vi "FromMonitorZoomOffset.vi"(8 "error in":errorcluster, 10 "Size":T1, 11 "Offset":T1) -> ()   [LabVIEW 2016]
uses:
  <vilib>/Utility/miscctls.llb/LVPointDoubleTypeDef.ctl
  Course Project/support/Message Queue/Message Cluster.ctl
  Course Project/support/Message Queue/Message Queue.lvlib
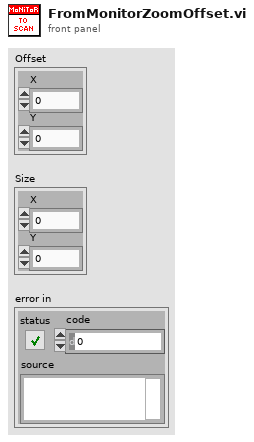
[diagram p1: front panel]
types:
  T1 = typedef "LVPointDoubleTypeDef.ctl" = cluster{"X":dbl, "Y":dbl}
  T2 = typedef "Message Queue.lvlib/Message Cluster.ctl" = cluster{"Message":string, "Données de message":variant}
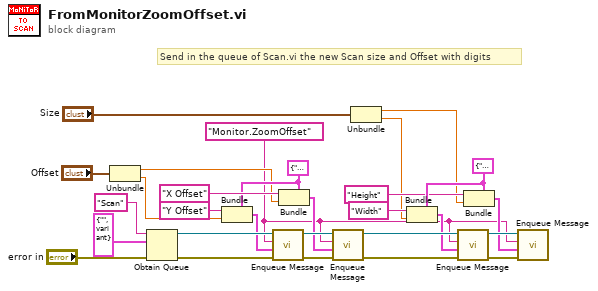
[diagram p0: block diagram]
diagram:
  w28 = cluster{"ControlName":string, "Value":dbl} {"ControlName"="", "Value"=0.0} ("Data")
  w9 = cluster{"ControlName":string, "Value":dbl} {"ControlName"="", "Value"=0.0} ("Data")
  w5 = "Monitor.ZoomOffset" ("Message")
  # "Send in the queue of Scan.vi the new Scan size and Offset with digits"
  n1 = Unbundle("Offset") -> ("X"=w6:dbl, "Y"=w10:dbl)
  n2 = Obtain Queue(name (unnamed)="Scan" ("QueueName"), element data type=T2 {"Message"="", "Données de message"=variant} ("Cluster Message"), error in (no error)="error in") -> (queue out=w26:refnum<queue>, error out=w15:errorcluster)  [unwired: 2 in, 1 out]
  n3 = Bundle(cluster=w9, "ControlName"="Y Offset" ("Message"), "Value"=w10) -> (w8:cluster{"ControlName":string, "Value":dbl})
  n4 = call "Enqueue Message.vi"("error in"=w15, "Data"=w8, "Message"=w5, "Queue"=w26) -> ("error out"=w16:errorcluster, "Queue dup."=w24:refnum<queue>)  [unwired: 6 in]
  n5 = Bundle(cluster=w9, "ControlName"="X Offset" ("Message"), "Value"=w6) -> (w7:cluster{"ControlName":string, "Value":dbl})
  n6 = call "Enqueue Message.vi"("error in"=w16, "Data"=w7, "Message"=w5, "Queue"=w24) -> ("error out"=w22:errorcluster, "Queue dup."=w25:refnum<queue>)  [unwired: 6 in]
  n7 = Unbundle("Size") -> ("X"=w4:dbl, "Y"=w3:dbl)
  n8 = Bundle(cluster=w28, "ControlName"="Width" ("Message"), "Value"=w3) -> (w20:cluster{"ControlName":string, "Value":dbl})
  n9 = call "Enqueue Message.vi"("error in"=w22, "Data"=w20, "Message"=w5, "Queue"=w25) -> ("error out"=w17:errorcluster, "Queue dup."=w27:refnum<queue>)  [unwired: 6 in]
  n10 = Bundle(cluster=w28, "ControlName"="Height" ("Message"), "Value"=w4) -> (w21:cluster{"ControlName":string, "Value":dbl})
  n11 = call "Enqueue Message.vi"("error in"=w17, "Data"=w21, "Message"=w5, "Queue"=w27) -> ()  [unwired: 6 in, 2 out]
